vi "save_configuration.vi"(0 "input cluster":T1) -> ()   [LabVIEW 2010]
uses:
  <vilib>/Utility/xml.llb/Write to XML File(string).vi
panel:
  out "xml string":string
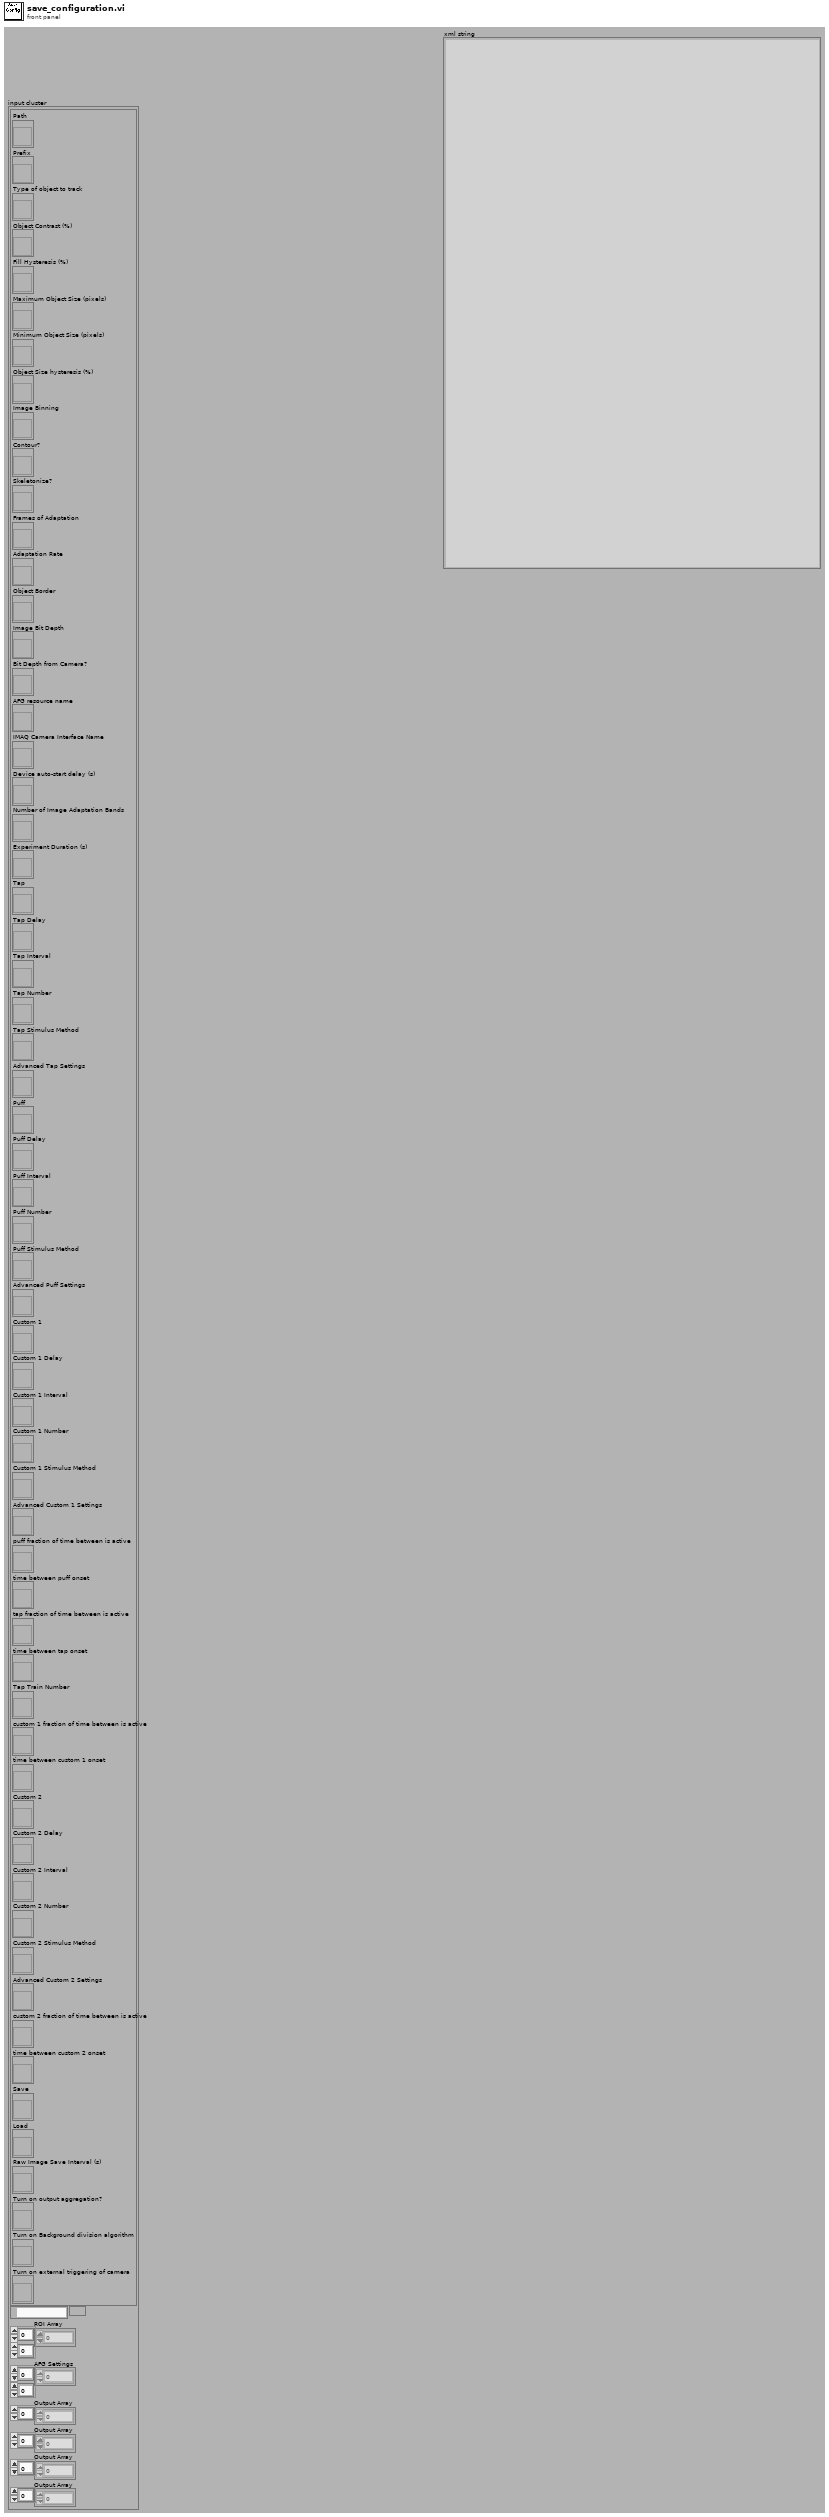
[diagram p1: front panel]
types:
  T1 = cluster{cluster{"Path":refnum<vi>, "Prefix":refnum<vi>, "Type of object to track":refnum<vi>, "Object Contrast (%)":refnum<vi>, "Fill Hysteresis (%)":refnum<vi>, "Maximum Object Size (pixels)":refnum<vi>, "Minimum Object Size (pixels)":refnum<vi>, "Object Size hysteresis (%)":refnum<vi>, "Image Binning":refnum<vi>, "Contour?":refnum<vi>, "Skeletonize?":refnum<vi>, "Frames of Adaptation":refnum<vi>, "Adaptation Rate":refnum<vi>, "Object Border":refnum<vi>, "Image Bit Depth":refnum<vi>, "Bit Depth from Camera?":refnum<vi>, "AFG resource name":refnum<vi>, "IMAQ Camera Interface Name":refnum<vi>, "Device auto-start delay (s)":refnum<vi>, "Number of Image Adaptation Bands":refnum<vi>, "Experiment Duration (s)":refnum<vi>, "Tap":refnum<vi>, "Tap Delay":refnum<vi>, "Tap Interval":refnum<vi>, "Tap Number":refnum<vi>, "Tap Stimulus Method":refnum<vi>, "Advanced Tap Settings":refnum<vi>, "Puff":refnum<vi>, "Puff Delay":refnum<vi>, "Puff Interval":refnum<vi>, "Puff Number":refnum<vi>, "Puff Stimulus Method":refnum<vi>, "Advanced Puff Settings":refnum<vi>, "Custom 1":refnum<vi>, "Custom 1 Delay":refnum<vi>, "Custom 1 Interval":refnum<vi>, "Custom 1 Number":refnum<vi>, "Custom 1 Stimulus Method":refnum<vi>, "Advanced Custom 1 Settings":refnum<vi>, "puff fraction of time between is active":refnum<vi>, "time between puff onset":refnum<vi>, "tap fraction of time between is active":refnum<vi>, "time between tap onset":refnum<vi>, "Tap Train Number":refnum<vi>, "custom 1 fraction of time between is active":refnum<vi>, "time between custom 1 onset":refnum<vi>, "Custom 2":refnum<vi>, "Custom 2 Delay":refnum<vi>, "Custom 2 Interval":refnum<vi>, "Custom 2 Number":refnum<vi>, "Custom 2 Stimulus Method":refnum<vi>, "Advanced Custom 2 Settings":refnum<vi>, "custom 2 fraction of time between is active":refnum<vi>, "time between custom 2 onset":refnum<vi>, "Save":refnum<vi>, "Load":refnum<vi>, "Raw Image Save Interval (s)":refnum<vi>, "Turn on output aggregation?":refnum<vi>, "Turn on Background division algorithm":refnum<vi>, "Turn on external triggering of camera":refnum<vi>}, path, "ROI Array":dbl[][], "AFG Settings":dbl[][], "Output Array":dbl[], "Output Array":dbl[], "Output Array":dbl[], "Output Array":dbl[]}
  T2 = cluster{"Path":refnum<vi>, "Prefix":refnum<vi>, "Type of object to track":refnum<vi>, "Object Contrast (%)":refnum<vi>, "Fill Hysteresis (%)":refnum<vi>, "Maximum Object Size (pixels)":refnum<vi>, "Minimum Object Size (pixels)":refnum<vi>, "Object Size hysteresis (%)":refnum<vi>, "Image Binning":refnum<vi>, "Contour?":refnum<vi>, "Skeletonize?":refnum<vi>, "Frames of Adaptation":refnum<vi>, "Adaptation Rate":refnum<vi>, "Object Border":refnum<vi>, "Image Bit Depth":refnum<vi>, "Bit Depth from Camera?":refnum<vi>, "AFG resource name":refnum<vi>, "IMAQ Camera Interface Name":refnum<vi>, "Device auto-start delay (s)":refnum<vi>, "Number of Image Adaptation Bands":refnum<vi>, "Experiment Duration (s)":refnum<vi>, "Tap":refnum<vi>, "Tap Delay":refnum<vi>, "Tap Interval":refnum<vi>, "Tap Number":refnum<vi>, "Tap Stimulus Method":refnum<vi>, "Advanced Tap Settings":refnum<vi>, "Puff":refnum<vi>, "Puff Delay":refnum<vi>, "Puff Interval":refnum<vi>, "Puff Number":refnum<vi>, "Puff Stimulus Method":refnum<vi>, "Advanced Puff Settings":refnum<vi>, "Custom 1":refnum<vi>, "Custom 1 Delay":refnum<vi>, "Custom 1 Interval":refnum<vi>, "Custom 1 Number":refnum<vi>, "Custom 1 Stimulus Method":refnum<vi>, "Advanced Custom 1 Settings":refnum<vi>, "puff fraction of time between is active":refnum<vi>, "time between puff onset":refnum<vi>, "tap fraction of time between is active":refnum<vi>, "time between tap onset":refnum<vi>, "Tap Train Number":refnum<vi>, "custom 1 fraction of time between is active":refnum<vi>, "time between custom 1 onset":refnum<vi>, "Custom 2":refnum<vi>, "Custom 2 Delay":refnum<vi>, "Custom 2 Interval":refnum<vi>, "Custom 2 Number":refnum<vi>, "Custom 2 Stimulus Method":refnum<vi>, "Advanced Custom 2 Settings":refnum<vi>, "custom 2 fraction of time between is active":refnum<vi>, "time between custom 2 onset":refnum<vi>, "Save":refnum<vi>, "Load":refnum<vi>, "Raw Image Save Interval (s)":refnum<vi>, "Turn on output aggregation?":refnum<vi>, "Turn on Background division algorithm":refnum<vi>, "Turn on external triggering of camera":refnum<vi>}
  T3 = cluster{"Label.Text":string, "Value":refnum<k15>}
  T4 = cluster{cluster{"Label.Text":string, "Value":path}, cluster{"Label.Text":string, "Value":string}, cluster{"Label.Text":string, "Value":bool}, cluster{"Label.Text":string, "Value":dbl}, cluster{"Label.Text":string, "Value":dbl}, cluster{"Label.Text":string, "Value":i32}, cluster{"Label.Text":string, "Value":i32}, cluster{"Label.Text":string, "Value":dbl}, cluster{"Label.Text":string, "Value":u16}, cluster{"Label.Text":string, "Value":bool}, cluster{"Label.Text":string, "Value":bool}, cluster{"Label.Text":string, "Value":i32}, cluster{"Label.Text":string, "Value":i32}, cluster{"Label.Text":string, "Value":i32}, cluster{"Label.Text":string, "Value":u32}, cluster{"Label.Text":string, "Value":bool}, cluster{"Label.Text":string, "Value":refnum<k15>}, cluster{"Label.Text":string, "Value":string}, cluster{"Label.Text":string, "Value":i32}, cluster{"Label.Text":string, "Value":i32}, cluster{"Label.Text":string, "Value":dbl}, cluster{"Label.Text":string, "Value":bool}, cluster{"Label.Text":string, "Value":dbl}, cluster{"Label.Text":string, "Value":dbl}, cluster{"Label.Text":string, "Value":i32}, cluster{"Label.Text":string, "Value":u16}, cluster{"Label.Text":string, "Value":bool}, cluster{"Label.Text":string, "Value":dbl}, cluster{"Label.Text":string, "Value":dbl}, cluster{"Label.Text":string, "Value":i32}, cluster{"Label.Text":string, "Value":u16}, cluster{"Label.Text":string, "Value":bool}, cluster{"Label.Text":string, "Value":dbl}, cluster{"Label.Text":string, "Value":dbl}, cluster{"Label.Text":string, "Value":i32}, cluster{"Label.Text":string, "Value":u16}, cluster{"Label.Text":string, "Value":sgl[][]}, cluster{"Label.Text":string, "Value":i32[][]}, cluster{"Label.Text":string, "Value":sgl[][]}, cluster{"Label.Text":string, "Value":i32[][]}, cluster{"Label.Text":string, "Value":i32[][]}, cluster{"Label.Text":string, "Value":sgl[][]}, cluster{"Label.Text":string, "Value":i32[][]}, cluster{"Label.Text":string, "Value":bool}, cluster{"Label.Text":string, "Value":dbl}, cluster{"Label.Text":string, "Value":dbl}, cluster{"Label.Text":string, "Value":i32}, cluster{"Label.Text":string, "Value":u16}, cluster{"Label.Text":string, "Value":sgl[][]}, cluster{"Label.Text":string, "Value":i32[][]}, cluster{"Label.Text":string, "Value":dbl}, cluster{"Label.Text":string, "Value":bool}, cluster{"Label.Text":string, "Value":bool}, cluster{"Label.Text":string, "Value":bool}, "ROI Array":dbl[][], "AFG Settings":dbl[][], "Output Array":dbl[], "Output Array":dbl[], "Output Array":dbl[], "Output Array":dbl[]}
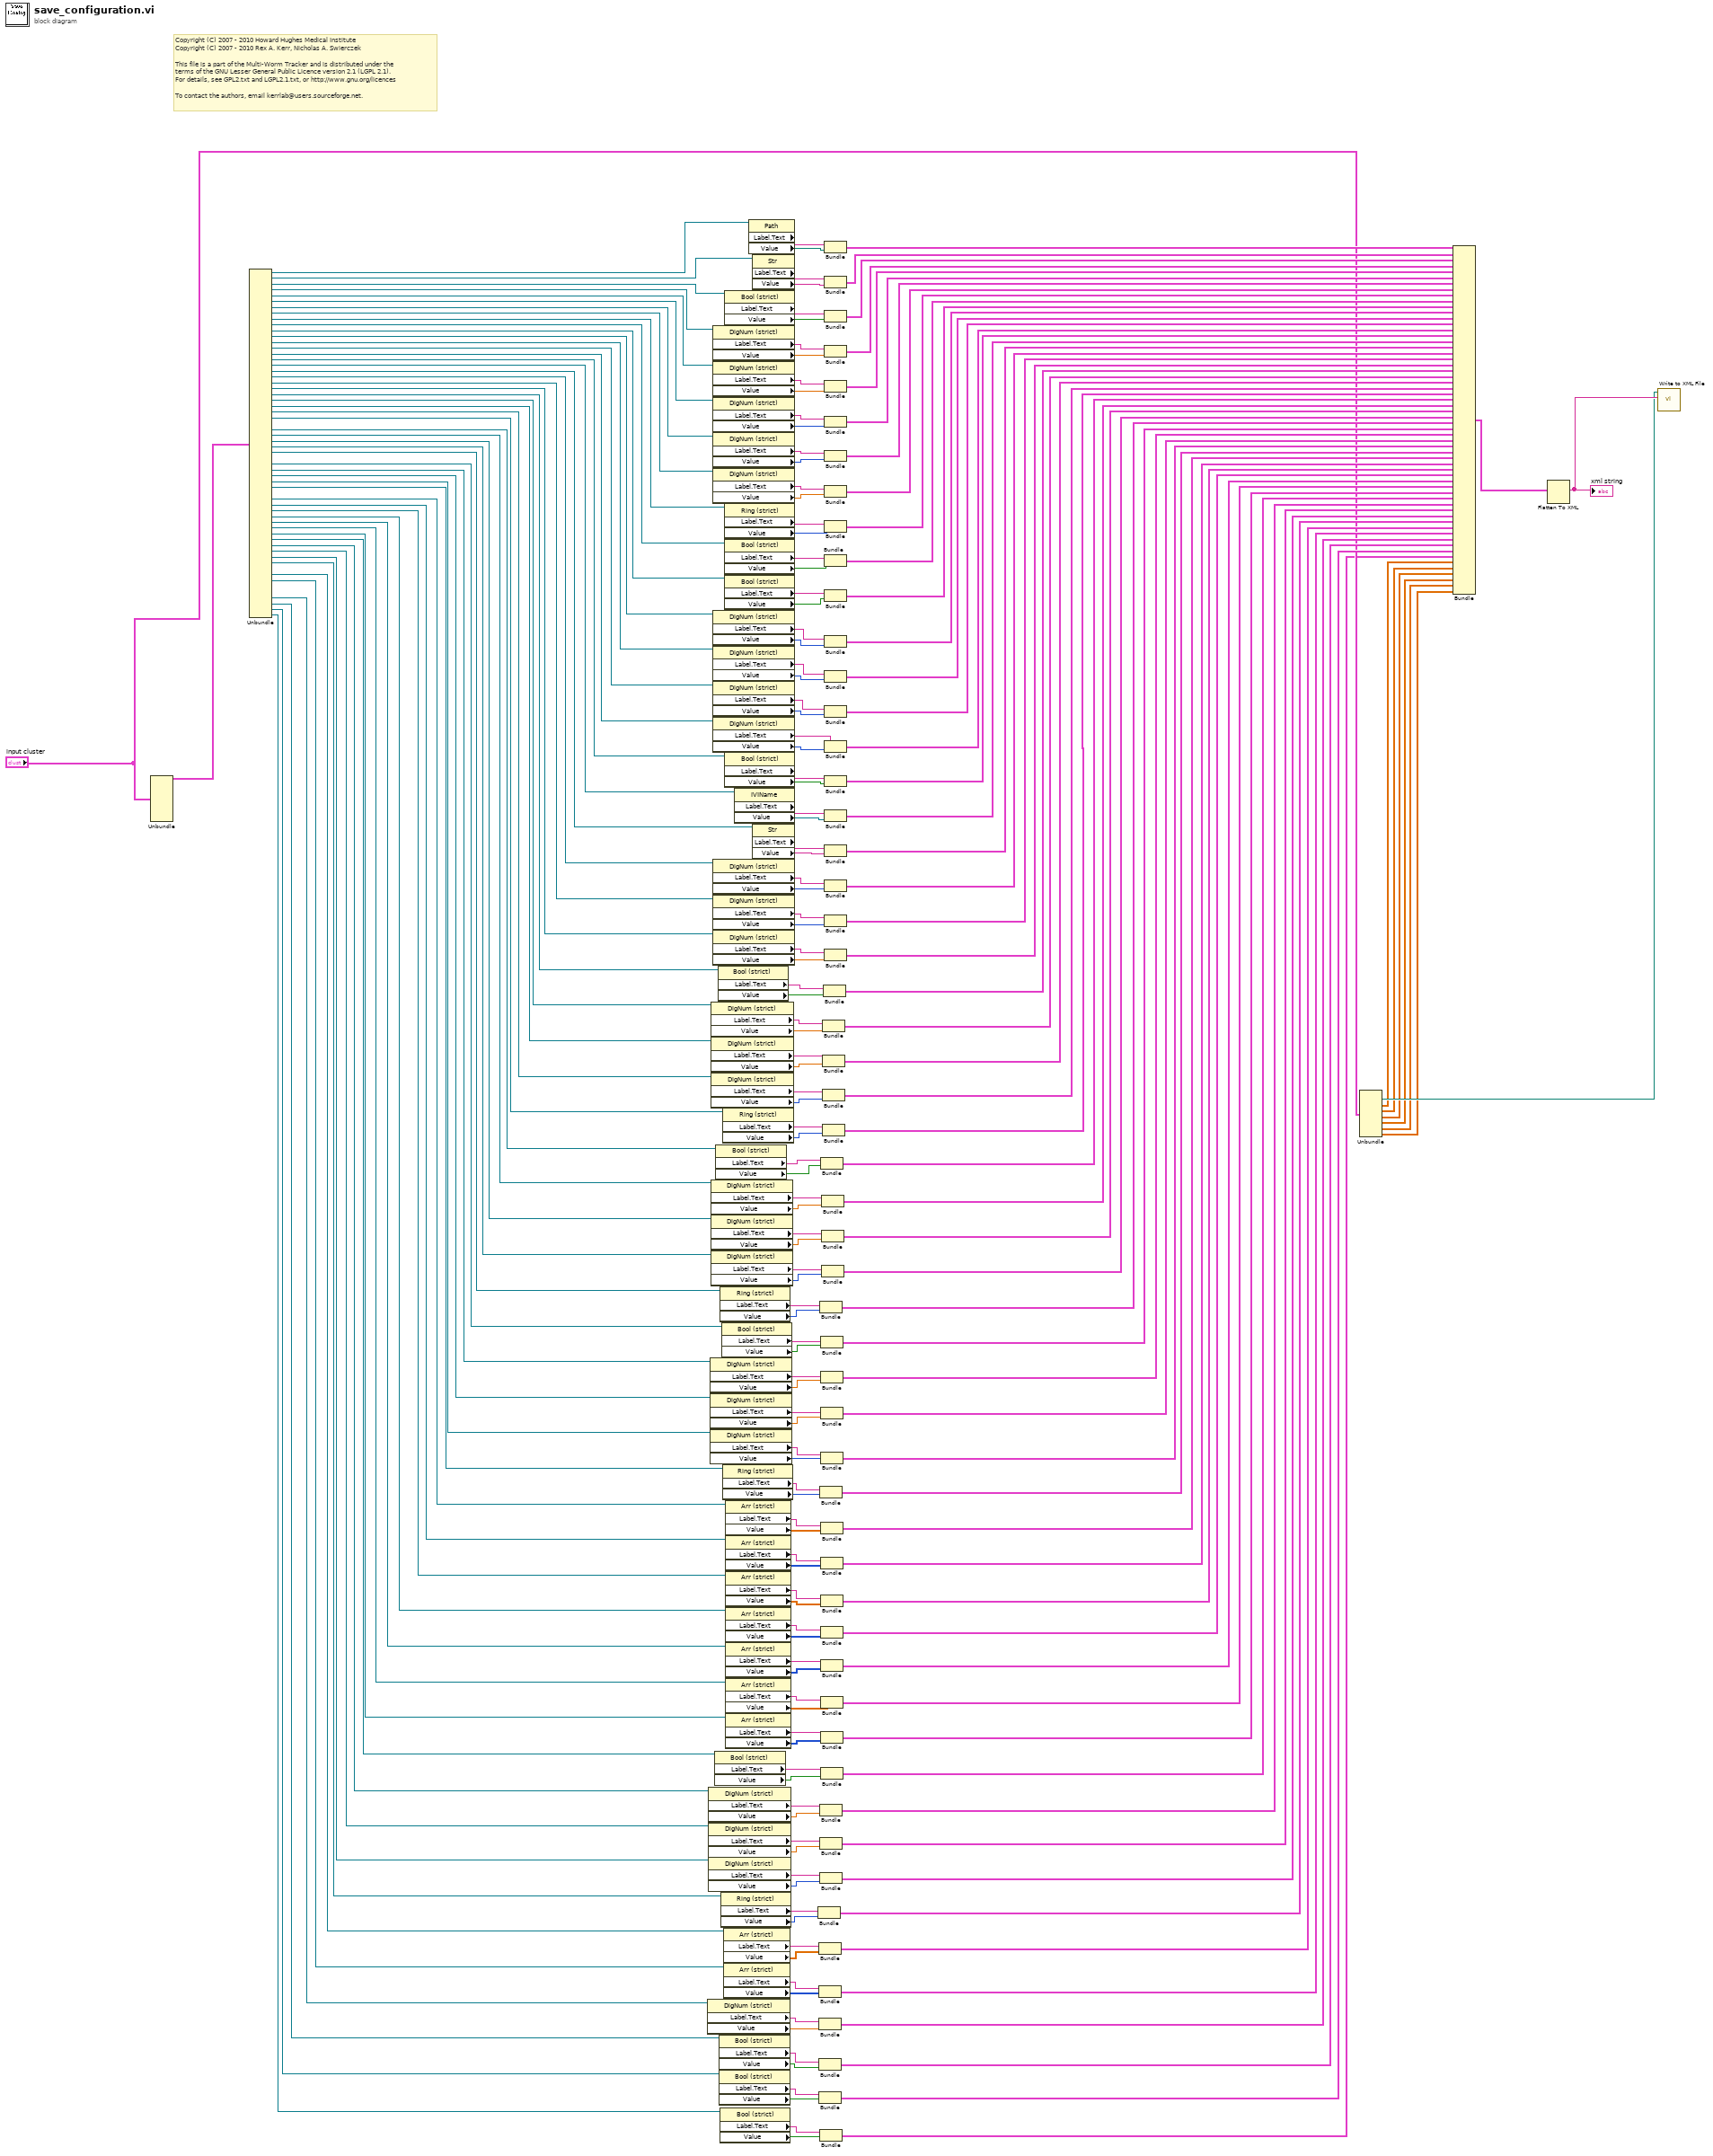
[diagram p0: block diagram]
diagram:
  # "Copyright (C) 2007 - 2010 Howard Hughes Medical Institute\nCopyright (C) 2007 - 2010 Rex A. Kerr, Nicholas A. Swierczek\n \nThis file is a part of the Multi-Worm Tracker and is distributed under the\nterms of the GNU Lesser General Public Licence version 2.1 (LGPL 2.1).\nFor details, see GPL2.txt and LGPL2.1.txt, or http://www.gnu.org/licences\n \nTo contact the authors, email kerrlab@users.sourceforge.net."
  n1 = Unbundle("input cluster") -> (w86:T2)  [unwired: 7 out]
  n2 = Unbundle(w86) -> ("Path"=w227:refnum<vi>, "Prefix"=w226:refnum<vi>, "Type of object to track"=w225:refnum<vi>, "Object Contrast (%)"=w224:refnum<vi>, "Fill Hysteresis (%)"=w223:refnum<vi>, "Maximum Object Size (pixels)"=w222:refnum<vi>, "Minimum Object Size (pixels)"=w221:refnum<vi>, "Object Size hysteresis (%)"=w220:refnum<vi>, "Image Binning"=w219:refnum<vi>, "Contour?"=w218:refnum<vi>, "Skeletonize?"=w217:refnum<vi>, "Frames of Adaptation"=w216:refnum<vi>, "Adaptation Rate"=w215:refnum<vi>, "Object Border"=w214:refnum<vi>, "Image Bit Depth"=w213:refnum<vi>, "Bit Depth from Camera?"=w212:refnum<vi>, "AFG resource name"=w211:refnum<vi>, "IMAQ Camera Interface Name"=w210:refnum<vi>, "Device auto-start delay (s)"=w209:refnum<vi>, "Number of Image Adaptation Bands"=w208:refnum<vi>, "Experiment Duration (s)"=w207:refnum<vi>, "Tap"=w82:refnum<vi>, "Tap Delay"=w206:refnum<vi>, "Tap Interval"=w205:refnum<vi>, "Tap Number"=w204:refnum<vi>, "Tap Stimulus Method"=w203:refnum<vi>, "Puff"=w79:refnum<vi>, "Puff Delay"=w202:refnum<vi>, "Puff Interval"=w201:refnum<vi>, "Puff Number"=w200:refnum<vi>, "Puff Stimulus Method"=w76:refnum<vi>, "Custom 1"=w199:refnum<vi>, "Custom 1 Delay"=w198:refnum<vi>, "Custom 1 Interval"=w197:refnum<vi>, "Custom 1 Number"=w196:refnum<vi>, "Custom 1 Stimulus Method"=w67:refnum<vi>, "puff fraction of time between is active"=w195:refnum<vi>, "time between puff onset"=w194:refnum<vi>, "tap fraction of time between is active"=w193:refnum<vi>, "time between tap onset"=w192:refnum<vi>, "Tap Train Number"=w191:refnum<vi>, "custom 1 fraction of time between is active"=w190:refnum<vi>, "time between custom 1 onset"=w189:refnum<vi>, "Custom 2"=w71:refnum<vi>, "Custom 2 Delay"=w188:refnum<vi>, "Custom 2 Interval"=w187:refnum<vi>, "Custom 2 Number"=w186:refnum<vi>, "Custom 2 Stimulus Method"=w73:refnum<vi>, "custom 2 fraction of time between is active"=w185:refnum<vi>, "time between custom 2 onset"=w184:refnum<vi>, "Raw Image Save Interval (s)"=w183:refnum<vi>, "Turn on output aggregation?"=w182:refnum<vi>, "Turn on Background division algorithm"=w181:refnum<vi>, "Turn on external triggering of camera"=w8:refnum<vi>)  [unwired: 6 out]
  n3 = property class="DigNum (strict)"(reference=w183) -> ("Label.Text"=w92:string, "Value"=w91:dbl)  [unwired: 1 in, 2 out]
  n4 = property class="DigNum (strict)"(reference=w188) -> ("Label.Text"=w102:string, "Value"=w101:dbl)  [unwired: 1 in, 2 out]
  n5 = property class="DigNum (strict)"(reference=w187) -> ("Label.Text"=w100:string, "Value"=w99:dbl)  [unwired: 1 in, 2 out]
  n6 = property class="DigNum (strict)"(reference=w186) -> ("Label.Text"=w98:string, "Value"=w97:i32)  [unwired: 1 in, 2 out]
  n7 = property class="DigNum (strict)"(reference=w198) -> ("Label.Text"=w122:string, "Value"=w121:dbl)  [unwired: 1 in, 2 out]
  n8 = property class="DigNum (strict)"(reference=w197) -> ("Label.Text"=w120:string, "Value"=w119:dbl)  [unwired: 1 in, 2 out]
  n9 = property class="DigNum (strict)"(reference=w196) -> ("Label.Text"=w118:string, "Value"=w117:i32)  [unwired: 1 in, 2 out]
  n10 = property class="DigNum (strict)"(reference=w202) -> ("Label.Text"=w130:string, "Value"=w129:dbl)  [unwired: 1 in, 2 out]
  n11 = property class="DigNum (strict)"(reference=w201) -> ("Label.Text"=w128:string, "Value"=w127:dbl)  [unwired: 1 in, 2 out]
  n12 = property class="DigNum (strict)"(reference=w200) -> ("Label.Text"=w126:string, "Value"=w125:i32)  [unwired: 1 in, 2 out]
  n13 = property class="DigNum (strict)"(reference=w206) -> ("Label.Text"=w138:string, "Value"=w137:dbl)  [unwired: 1 in, 2 out]
  n14 = property class="DigNum (strict)"(reference=w205) -> ("Label.Text"=w136:string, "Value"=w135:dbl)  [unwired: 1 in, 2 out]
  n15 = property class="DigNum (strict)"(reference=w204) -> ("Label.Text"=w134:string, "Value"=w133:i32)  [unwired: 1 in, 2 out]
  n16 = property class="DigNum (strict)"(reference=w224) -> ("Label.Text"=w174:string, "Value"=w173:dbl)  [unwired: 1 in, 2 out]
  n17 = property class="DigNum (strict)"(reference=w223) -> ("Label.Text"=w172:string, "Value"=w171:dbl)  [unwired: 1 in, 2 out]
  n18 = property class="DigNum (strict)"(reference=w222) -> ("Label.Text"=w170:string, "Value"=w169:i32)  [unwired: 1 in, 2 out]
  n19 = property class="DigNum (strict)"(reference=w221) -> ("Label.Text"=w168:string, "Value"=w167:i32)  [unwired: 1 in, 2 out]
  n20 = property class="DigNum (strict)"(reference=w220) -> ("Label.Text"=w166:string, "Value"=w165:dbl)  [unwired: 1 in, 2 out]
  n21 = property class="DigNum (strict)"(reference=w216) -> ("Label.Text"=w158:string, "Value"=w157:i32)  [unwired: 1 in, 2 out]
  n22 = property class="DigNum (strict)"(reference=w215) -> ("Label.Text"=w156:string, "Value"=w155:i32)  [unwired: 1 in, 2 out]
  n23 = property class="DigNum (strict)"(reference=w214) -> ("Label.Text"=w154:string, "Value"=w153:i32)  [unwired: 1 in, 2 out]
  n24 = property class="DigNum (strict)"(reference=w213) -> ("Label.Text"=w152:string, "Value"=w151:u32)  [unwired: 1 in, 2 out]
  n25 = property class="DigNum (strict)"(reference=w209) -> ("Label.Text"=w144:string, "Value"=w143:i32)  [unwired: 1 in, 2 out]
  n26 = property class="DigNum (strict)"(reference=w208) -> ("Label.Text"=w142:string, "Value"=w141:i32)  [unwired: 1 in, 2 out]
  n27 = property class="DigNum (strict)"(reference=w207) -> ("Label.Text"=w140:string, "Value"=w139:dbl)  [unwired: 1 in, 2 out]
  n28 = property class="Bool (strict)"(reference=w71) -> ("Label.Text"=w72:string, "Value"=w70:bool)  [unwired: 1 in, 2 out]
  n29 = property class="Bool (strict)"(reference=w79) -> ("Label.Text"=w81:string, "Value"=w80:bool)  [unwired: 1 in, 2 out]
  n30 = property class="Bool (strict)"(reference=w82) -> ("Label.Text"=w84:string, "Value"=w83:bool)  [unwired: 1 in, 2 out]
  n31 = property class="Bool (strict)"(reference=w182) -> ("Label.Text"=w90:string, "Value"=w89:bool)  [unwired: 1 in, 2 out]
  n32 = property class="Bool (strict)"(reference=w181) -> ("Label.Text"=w88:string, "Value"=w87:bool)  [unwired: 1 in, 2 out]
  n33 = property class="Ring (strict)"(reference=w76) -> ("Label.Text"=w77:string, "Value"=w78:u16)  [unwired: 1 in, 2 out]
  n34 = property class="Bool (strict)"(reference=w8) -> ("Label.Text"=w9:string, "Value"=w10:bool)  [unwired: 1 in, 2 out]
  n35 = property class="Ring (strict)"(reference=w73) -> ("Label.Text"=w74:string, "Value"=w75:u16)  [unwired: 1 in, 2 out]
  n36 = property class="Bool (strict)"(reference=w199) -> ("Label.Text"=w124:string, "Value"=w123:bool)  [unwired: 1 in, 2 out]
  n37 = property class="Ring (strict)"(reference=w67) -> ("Label.Text"=w68:string, "Value"=w69:u16)  [unwired: 1 in, 2 out]
  n38 = property class="Ring (strict)"(reference=w203) -> ("Label.Text"=w132:string, "Value"=w131:u16)  [unwired: 1 in, 2 out]
  n39 = property class="Arr (strict)"(reference=w185) -> ("Label.Text"=w96:string, "Value"=w95:sgl[][])  [unwired: 1 in, 2 out]
  n40 = property class="Arr (strict)"(reference=w184) -> ("Label.Text"=w94:string, "Value"=w93:i32[][])  [unwired: 1 in, 2 out]
  n41 = property class="Bool (strict)"(reference=w225) -> ("Label.Text"=w176:string, "Value"=w175:bool)  [unwired: 1 in, 2 out]
  n42 = property class="Ring (strict)"(reference=w219) -> ("Label.Text"=w164:string, "Value"=w163:u16)  [unwired: 1 in, 2 out]
  n43 = property class="Bool (strict)"(reference=w218) -> ("Label.Text"=w162:string, "Value"=w161:bool)  [unwired: 1 in, 2 out]
  n44 = property class="Bool (strict)"(reference=w217) -> ("Label.Text"=w160:string, "Value"=w159:bool)  [unwired: 1 in, 2 out]
  n45 = property class="Bool (strict)"(reference=w212) -> ("Label.Text"=w150:string, "Value"=w149:bool)  [unwired: 1 in, 2 out]
  n46 = property class="Arr (strict)"(reference=w195) -> ("Label.Text"=w116:string, "Value"=w115:sgl[][])  [unwired: 1 in, 2 out]
  n47 = property class="Arr (strict)"(reference=w194) -> ("Label.Text"=w114:string, "Value"=w113:i32[][])  [unwired: 1 in, 2 out]
  n48 = property class="Arr (strict)"(reference=w193) -> ("Label.Text"=w112:string, "Value"=w111:sgl[][])  [unwired: 1 in, 2 out]
  n49 = property class="Arr (strict)"(reference=w192) -> ("Label.Text"=w110:string, "Value"=w109:i32[][])  [unwired: 1 in, 2 out]
  n50 = property class="Arr (strict)"(reference=w191) -> ("Label.Text"=w108:string, "Value"=w107:i32[][])  [unwired: 1 in, 2 out]
  n51 = property class="Arr (strict)"(reference=w190) -> ("Label.Text"=w106:string, "Value"=w105:sgl[][])  [unwired: 1 in, 2 out]
  n52 = property class="Arr (strict)"(reference=w189) -> ("Label.Text"=w104:string, "Value"=w103:i32[][])  [unwired: 1 in, 2 out]
  n53 = property class="IVIName"(reference=w211) -> ("Label.Text"=w148:string, "Value"=w147:refnum<k15>)  [unwired: 1 in, 2 out]
  n54 = property class="Path"(reference=w227) -> ("Label.Text"=w180:string, "Value"=w179:path)  [unwired: 1 in, 2 out]
  n55 = property class="Str"(reference=w226) -> ("Label.Text"=w178:string, "Value"=w177:string)  [unwired: 1 in, 2 out]
  n56 = property class="Str"(reference=w210) -> ("Label.Text"=w146:string, "Value"=w145:string)  [unwired: 1 in, 2 out]
  n57 = Bundle("Label.Text"=w74, "Value"=w75) -> (w19:cluster{"Label.Text":string, "Value":u16})  [unwired: 1 in]
  n58 = Bundle("Label.Text"=w96, "Value"=w95) -> (w18:cluster{"Label.Text":string, "Value":sgl[][]})  [unwired: 1 in]
  n59 = Bundle("Label.Text"=w94, "Value"=w93) -> (w17:cluster{"Label.Text":string, "Value":i32[][]})  [unwired: 1 in]
  n60 = Bundle("Label.Text"=w92, "Value"=w91) -> (w16:cluster{"Label.Text":string, "Value":dbl})  [unwired: 1 in]
  n61 = Bundle("Label.Text"=w90, "Value"=w89) -> (w15:cluster{"Label.Text":string, "Value":bool})  [unwired: 1 in]
  n62 = Bundle("Label.Text"=w88, "Value"=w87) -> (w14:cluster{"Label.Text":string, "Value":bool})  [unwired: 1 in]
  n63 = Bundle("Label.Text"=w77, "Value"=w78) -> (w36:cluster{"Label.Text":string, "Value":u16})  [unwired: 1 in]
  n64 = Bundle("Label.Text"=w68, "Value"=w69) -> (w31:cluster{"Label.Text":string, "Value":u16})  [unwired: 1 in]
  n65 = Bundle("Label.Text"=w102, "Value"=w101) -> (w22:cluster{"Label.Text":string, "Value":dbl})  [unwired: 1 in]
  n66 = Bundle("Label.Text"=w100, "Value"=w99) -> (w21:cluster{"Label.Text":string, "Value":dbl})  [unwired: 1 in]
  n67 = Bundle("Label.Text"=w98, "Value"=w97) -> (w20:cluster{"Label.Text":string, "Value":i32})  [unwired: 1 in]
  n68 = Bundle("Label.Text"=w9, "Value"=w10) -> (w1:cluster{"Label.Text":string, "Value":bool})  [unwired: 1 in]
  n69 = Bundle("Label.Text"=w116, "Value"=w115) -> (w30:cluster{"Label.Text":string, "Value":sgl[][]})  [unwired: 1 in]
  n70 = Bundle("Label.Text"=w114, "Value"=w113) -> (w29:cluster{"Label.Text":string, "Value":i32[][]})  [unwired: 1 in]
  n71 = Bundle("Label.Text"=w112, "Value"=w111) -> (w28:cluster{"Label.Text":string, "Value":sgl[][]})  [unwired: 1 in]
  n72 = Bundle("Label.Text"=w110, "Value"=w109) -> (w27:cluster{"Label.Text":string, "Value":i32[][]})  [unwired: 1 in]
  n73 = Bundle("Label.Text"=w108, "Value"=w107) -> (w26:cluster{"Label.Text":string, "Value":i32[][]})  [unwired: 1 in]
  n74 = Bundle("Label.Text"=w106, "Value"=w105) -> (w25:cluster{"Label.Text":string, "Value":sgl[][]})  [unwired: 1 in]
  n75 = Bundle("Label.Text"=w104, "Value"=w103) -> (w24:cluster{"Label.Text":string, "Value":i32[][]})  [unwired: 1 in]
  n76 = Bundle("Label.Text"=w72, "Value"=w70) -> (w23:cluster{"Label.Text":string, "Value":bool})  [unwired: 1 in]
  n77 = Bundle("Label.Text"=w81, "Value"=w80) -> (w40:cluster{"Label.Text":string, "Value":bool})  [unwired: 1 in]
  n78 = Bundle("Label.Text"=w124, "Value"=w123) -> (w35:cluster{"Label.Text":string, "Value":bool})  [unwired: 1 in]
  n79 = Bundle("Label.Text"=w122, "Value"=w121) -> (w34:cluster{"Label.Text":string, "Value":dbl})  [unwired: 1 in]
  n80 = Bundle("Label.Text"=w120, "Value"=w119) -> (w33:cluster{"Label.Text":string, "Value":dbl})  [unwired: 1 in]
  n81 = Bundle("Label.Text"=w118, "Value"=w117) -> (w32:cluster{"Label.Text":string, "Value":i32})  [unwired: 1 in]
  n82 = Bundle("Label.Text"=w130, "Value"=w129) -> (w39:cluster{"Label.Text":string, "Value":dbl})  [unwired: 1 in]
  n83 = Bundle("Label.Text"=w128, "Value"=w127) -> (w38:cluster{"Label.Text":string, "Value":dbl})  [unwired: 1 in]
  n84 = Bundle("Label.Text"=w126, "Value"=w125) -> (w37:cluster{"Label.Text":string, "Value":i32})  [unwired: 1 in]
  n85 = Bundle("Label.Text"=w138, "Value"=w137) -> (w44:cluster{"Label.Text":string, "Value":dbl})  [unwired: 1 in]
  n86 = Bundle("Label.Text"=w136, "Value"=w135) -> (w43:cluster{"Label.Text":string, "Value":dbl})  [unwired: 1 in]
  n87 = Bundle("Label.Text"=w134, "Value"=w133) -> (w42:cluster{"Label.Text":string, "Value":i32})  [unwired: 1 in]
  n88 = Bundle("Label.Text"=w132, "Value"=w131) -> (w41:cluster{"Label.Text":string, "Value":u16})  [unwired: 1 in]
  n89 = Bundle("Label.Text"=w84, "Value"=w83) -> (w45:cluster{"Label.Text":string, "Value":bool})  [unwired: 1 in]
  n90 = Bundle("Label.Text"=w180, "Value"=w179) -> (w66:cluster{"Label.Text":string, "Value":path})  [unwired: 1 in]
  n91 = Bundle("Label.Text"=w178, "Value"=w177) -> (w65:cluster{"Label.Text":string, "Value":string})  [unwired: 1 in]
  n92 = Bundle("Label.Text"=w176, "Value"=w175) -> (w64:cluster{"Label.Text":string, "Value":bool})  [unwired: 1 in]
  n93 = Bundle("Label.Text"=w174, "Value"=w173) -> (w63:cluster{"Label.Text":string, "Value":dbl})  [unwired: 1 in]
  n94 = Bundle("Label.Text"=w172, "Value"=w171) -> (w62:cluster{"Label.Text":string, "Value":dbl})  [unwired: 1 in]
  n95 = Bundle("Label.Text"=w170, "Value"=w169) -> (w61:cluster{"Label.Text":string, "Value":i32})  [unwired: 1 in]
  n96 = Bundle("Label.Text"=w168, "Value"=w167) -> (w60:cluster{"Label.Text":string, "Value":i32})  [unwired: 1 in]
  n97 = Bundle("Label.Text"=w166, "Value"=w165) -> (w59:cluster{"Label.Text":string, "Value":dbl})  [unwired: 1 in]
  n98 = Bundle("Label.Text"=w164, "Value"=w163) -> (w58:cluster{"Label.Text":string, "Value":u16})  [unwired: 1 in]
  n99 = Bundle("Label.Text"=w162, "Value"=w161) -> (w57:cluster{"Label.Text":string, "Value":bool})  [unwired: 1 in]
  n100 = Bundle("Label.Text"=w160, "Value"=w159) -> (w56:cluster{"Label.Text":string, "Value":bool})  [unwired: 1 in]
  n101 = Bundle("Label.Text"=w158, "Value"=w157) -> (w55:cluster{"Label.Text":string, "Value":i32})  [unwired: 1 in]
  n102 = Bundle("Label.Text"=w156, "Value"=w155) -> (w54:cluster{"Label.Text":string, "Value":i32})  [unwired: 1 in]
  n103 = Bundle("Label.Text"=w154, "Value"=w153) -> (w53:cluster{"Label.Text":string, "Value":i32})  [unwired: 1 in]
  n104 = Bundle("Label.Text"=w152, "Value"=w151) -> (w52:cluster{"Label.Text":string, "Value":u32})  [unwired: 1 in]
  n105 = Bundle("Label.Text"=w150, "Value"=w149) -> (w51:cluster{"Label.Text":string, "Value":bool})  [unwired: 1 in]
  n106 = Bundle("Label.Text"=w148, "Value"=w147) -> (w50:T3)  [unwired: 1 in]
  n107 = Bundle("Label.Text"=w146, "Value"=w145) -> (w49:cluster{"Label.Text":string, "Value":string})  [unwired: 1 in]
  n108 = Bundle("Label.Text"=w144, "Value"=w143) -> (w48:cluster{"Label.Text":string, "Value":i32})  [unwired: 1 in]
  n109 = Bundle("Label.Text"=w142, "Value"=w141) -> (w47:cluster{"Label.Text":string, "Value":i32})  [unwired: 1 in]
  n110 = Bundle("Label.Text"=w140, "Value"=w139) -> (w46:cluster{"Label.Text":string, "Value":dbl})  [unwired: 1 in]
  n111 = Unbundle("input cluster") -> (w12:path, "ROI Array"=w2:dbl[][], "AFG Settings"=w3:dbl[][], "Output Array"=w4:dbl[], "Output Array"=w5:dbl[], "Output Array"=w6:dbl[], "Output Array"=w7:dbl[])  [unwired: 1 out]
  n112 = Bundle(w66, w65, w64, w63, w62, w61, w60, w59, w58, w57, w56, w55, w54, w53, w52, w51, w50, w49, w48, w47, w46, w45, w44, w43, w42, w41, w40, w39, w38, w37, w36, w35, w34, w33, w32, w31, w30, w29, w28, w27, w26, w25, w24, w23, w22, w21, w20, w19, w18, w17, w16, w15, w14, w1, "ROI Array"=w2, "AFG Settings"=w3, "Output Array"=w4, "Output Array"=w5, "Output Array"=w6, "Output Array"=w7) -> (w13:T4)  [unwired: 1 in]
  n113 = Flatten To XML(anything=w13) -> (xml string=w85:string)
  "xml string" <- w85
  n114 = call-poly <vilib>:"Write to XML File.vi"("XML Input"=w85, "XML File Path"=w12) -> ()  [unwired: 7 in, 3 out]
